vi "TS Shutdown.vi"(8 "error in (no error)":errorcluster, 11 "Auto UI in":refnum<class "Auto UI.lvclass">) -> (0 "error out":errorcluster, 3 "Auto UI out":refnum<class "Auto UI.lvclass">)   [LabVIEW 2023, in "GUI.lvlib" / "Auto UI.lvlib" / "Auto UI.lvclass"]
uses:
  Auto UI.lvclass
  Auto UI.lvclass/Auto UI.ctl
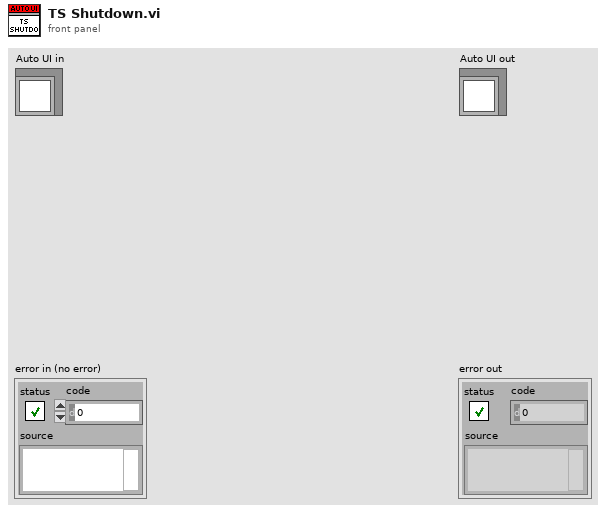
[diagram p1: front panel]
types:
  T1 = enum32{"invalid app kind", "Development System", "Run Time System", "Student Edition", "Embedded LabVIEW", "Evaluation", "Custom"}
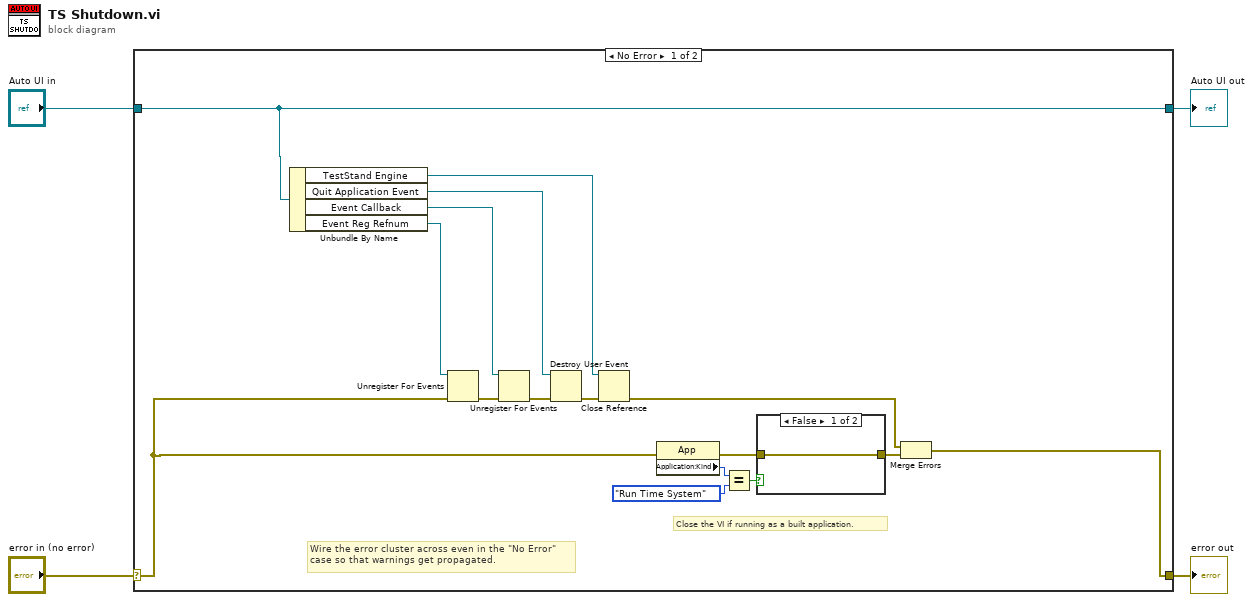
[diagram p0: block diagram]
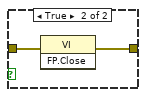
[diagram p2: hidden frame]
diagram:
  n1 = case shown="No Error" "error in (no error)" {
    selector: "error in (no error)" -> [w6 w25]
    tunnel: [w5 w25] -> w3
    tunnel: [w7 w24] -> w1
    tunnel: "Auto UI in" -> [w7 w24]
    frame No Error {
      # "Close the VI if running as a built application."
      # "Wire the error cluster across even in the \"No Error\"\ncase so that warnings get propagated."
      n2 = Unbundle By Name(w7) -> ("TestStand Engine"=w14:refnum<k7>, "Quit Application Event"=w16:refnum<user-event>, "Event Callback"=w18:refnum<k27>, "Event Reg Refnum"=w17:refnum<event-registration>)
      n3 = Unregister For Events(event registration refnum=w17, error in=w6) -> (error out=w19:errorcluster)
      n4 = Unregister For Events(event registration refnum=w18, error in=w19) -> (error out=w20:errorcluster)
      n5 = Destroy User Event(user event=w16, error in=w20) -> (error out=w15:errorcluster)
      n6 = Close Reference(reference=w14, error in (no error)=w15) -> (error out=w8:errorcluster)
      n7 = property class="App"(error in=w6) -> (error out=w10:errorcluster, "Application:Kind"=w12:T1)  [unwired: 1 in, 1 out]
      n8 = Equal?(x=w12, y=T1."Run Time System" ("Application:Kind")) -> (x = y?=w11:bool)
      n9 = case shown="False" w11 {
        tunnel: w10 -> [w21 w23]
        tunnel: [w21 w22] -> w9
        frame False {
        }
        frame True {
          n10 = invoke class="VI" method="FP.Close"(error in=w23) -> (error out=w22:errorcluster)  [unwired: 2 in, 2 out]
        }
      }
      n11 = Merge Errors(w8, w9) -> (w5:errorcluster)
    }
    frame Error {
    }
  }
  "error out" <- w3
  "Auto UI out" <- w1
